vi "P-612 Stage Engine.vi"(0 "Unique Notifier Name":string, 11 "COM Port":string[](array[string])) -> ()   [LabVIEW 2016]
uses:
  Stages Controls/Stage Status.ctl
  Stages Controls/Stage XY Control.ctl
  Stages Controls/Stage Notifier Element.ctl
  Stages Controls/Stage Actions.ctl
panel:
  in  "XY Control":T1={"Left"=FALSE, "Right"=FALSE, "Up"=FALSE, "Down"=FALSE, "Home"=FALSE, "StageStep"=enum."1", "Y"=0.0, "X"=0.0}
  in  "ReInitialize":bool
  in  "Error":bool
  out "Status":T2
  in  "QUIT":bool
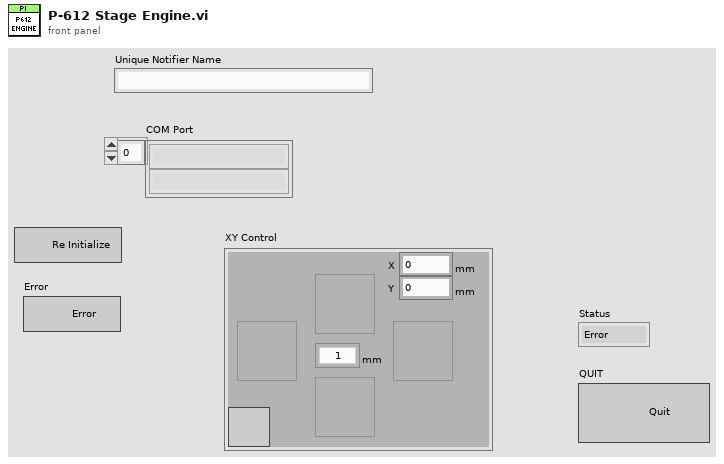
[diagram p1: front panel]
types:
  T1 = typedef "Stage XY Control.ctl" = cluster{"Left":bool, "Right":bool, "Up":bool, "Down":bool, "Home":bool, "StageStep":enum16{"0.01", "0.02", "0.05", "0.1", "0.5", "1", "2", "5", "10", "20", "50", "100", "500", "1000", "2000", "5000"}, "Y":dbl, "X":dbl}
  T2 = typedef "Stage Status.ctl" = enum16{"Error", "Abort", "Busy", "On Target"}
  T3 = typedef "Stage Actions.ctl" = enum16{"Get Position", "MVR", "MOVE", "HALT", "ONTARGET", "ERROR", "REFERENCE", "INIT", "VELOCITY", "STATUS", "EXIT", "HOME", "ZEROPOS", "NANOPOS", "ANALOG", "QUIT"}
  T4 = typedef "Stage Notifier Element.ctl" = cluster{"Action":T3, "Axis":bool[], "Setpoint":dbl[], "Velocity":dbl, "Cmd Recvd?":bool, "Position":dbl[], "Status":T2, "Misc":variant}
  T5 = cluster{"Left":bool, "Right":bool, "Up":bool, "Down":bool, "Home":bool, "StageStep":bool, "Y":bool, "X":bool}
  T6 = enum16{"0.01", "0.02", "0.05", "0.1", "0.5", "1", "2", "5", "10", "20", "50", "100", "500", "1000", "2000", "5000"}
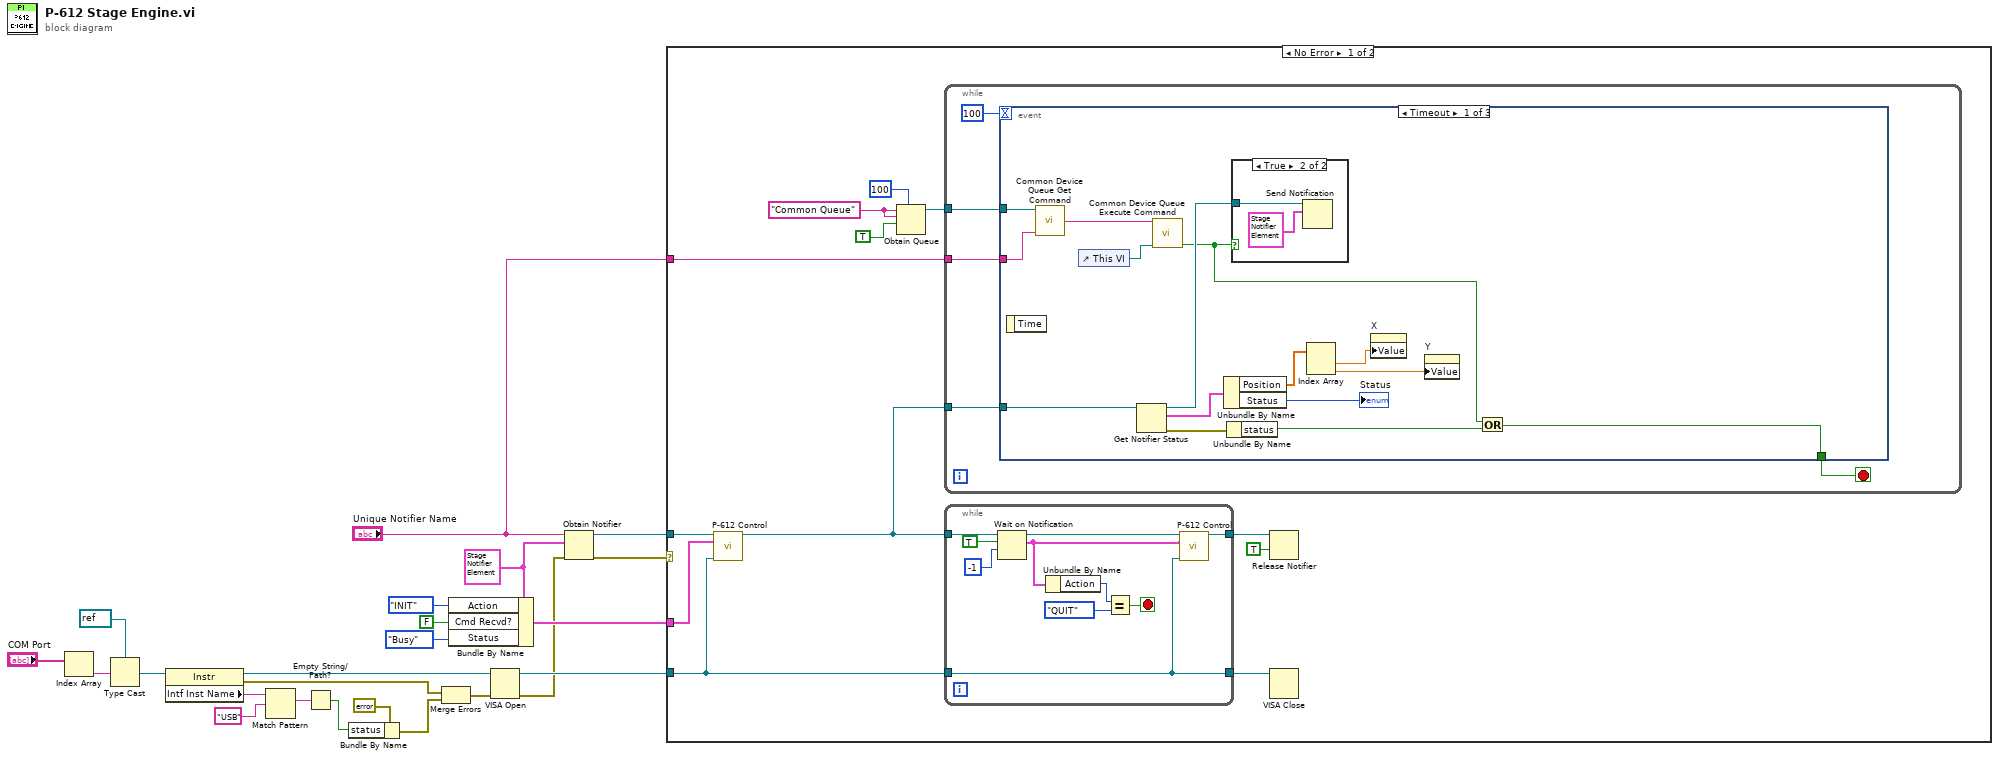
[diagram p0: block diagram]
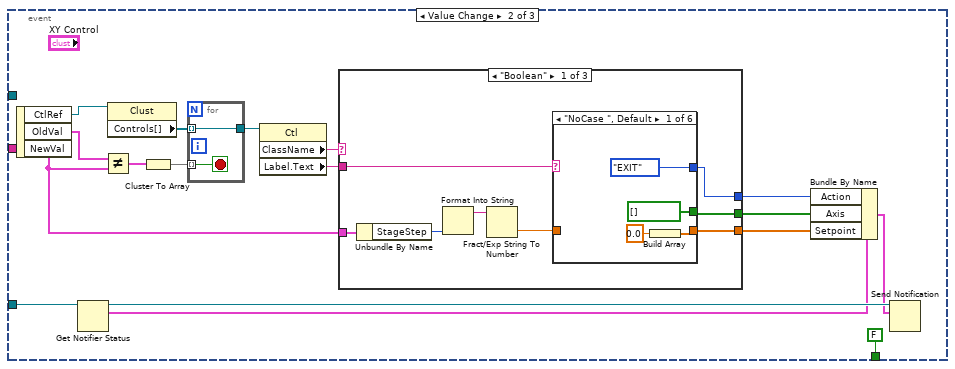
[diagram p3: hidden frame]
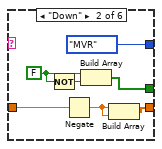
[diagram p4: hidden frame]
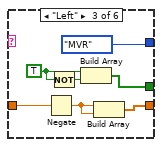
[diagram p5: hidden frame]
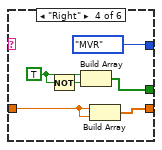
[diagram p6: hidden frame]
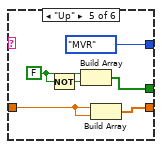
[diagram p7: hidden frame]
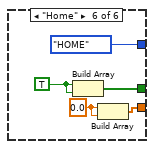
[diagram p8: hidden frame]
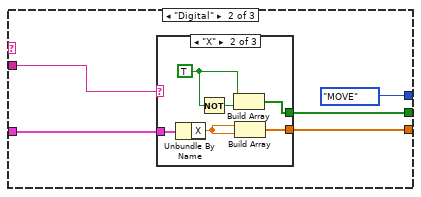
[diagram p9: hidden frame]
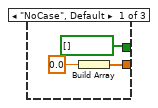
[diagram p10: hidden frame]
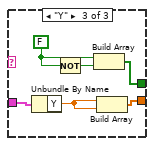
[diagram p11: hidden frame]
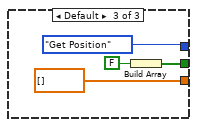
[diagram p12: hidden frame]
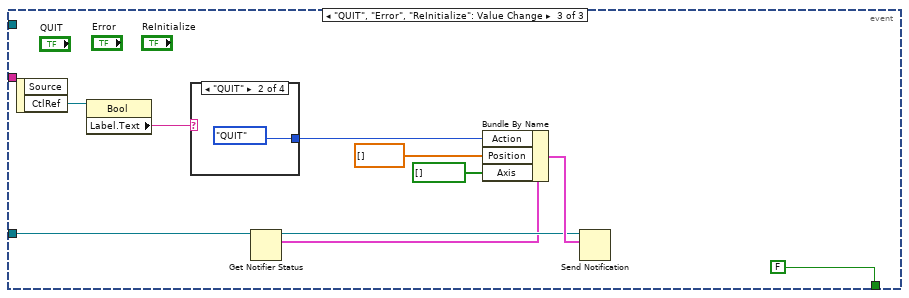
[diagram p13: hidden frame]
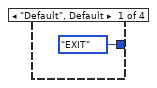
[diagram p14: hidden frame]
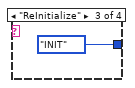
[diagram p15: hidden frame]
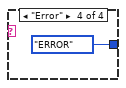
[diagram p16: hidden frame]
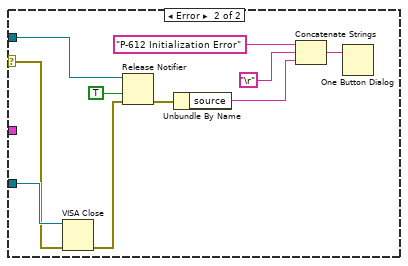
[diagram p17: hidden frame]
diagram:
  w9 = T4 {"Action"=enum."Get Position", "Axis"=[], "Setpoint"=[], "Velocity"=0.5, "Cmd Recvd?"=FALSE, "Position"=[], "Status"=enum."Abort", "Misc"=variant} ("Stage Status")
  n1 = Index Array(array="COM Port") -> (element=w18:string)  [unwired: 1 in]
  n2 = Type Cast(type=refnum<visa-resource-name> refnum ("reference out"), x=w18) -> (*(type *) &x=w16:refnum<visa-resource-name>)
  n3 = property class="Instr"(reference=w16) -> (reference out=w5:refnum<visa-resource-name>, error out=w13:errorcluster, "Intf Inst Name"=w21:string)  [unwired: 1 in]
  n4 = Match Pattern(string=w21, regular expression="USB") -> (match substring=w23:string)  [unwired: 1 in, 3 out]
  n5 = Empty String/Path?(string/path=w23) -> (empty?=w20:bool)
  n6 = Bundle By Name(cluster=errorcluster {"status"=FALSE, "code"=0, "source"=""} ("Error"), "status"=w20) -> (w14:errorcluster)
  n7 = Merge Errors(w13, w14) -> (w4:errorcluster)
  n8 = Bundle By Name(cluster=w9, "Action"=Stage_Actions."INIT", "Cmd Recvd?"=FALSE, "Status"=Stage_Status."Busy") -> (w6:T4)
  n9 = VISA Open(error in (no error)=w4, VISA resource name=w5) -> (VISA resource name=w3:refnum<visa-resource-name>, error out=w2:errorcluster)  [unwired: 3 in]
  n10 = Obtain Notifier(name (unnamed)="Unique Notifier Name", notification data type=w9, error in (no error)=w2) -> (notifier out=w7:refnum<notifier>, error out=w8:errorcluster)  [unwired: 1 in, 1 out]
  n11 = case shown="No Error" w8 {
    selector: w8 -> [_ w168]
    tunnel: w7 -> [w33 w170]
    tunnel: w6 -> [w32 _]
    tunnel: w3 -> [w31 w169]
    tunnel: "Unique Notifier Name" -> [w24 _]
    frame No Error {
      w27 = "Common Queue" ("Unique Notifier Name")
      n12 = call "P-612 Control.vi"("P-612 Notifier"=w33, "Stage Actions"=w32, "VISA In"=w31) -> ("P-612 Notifier (Dup)"=w26:refnum<notifier>)  [unwired: 12 in]
      n13 = Obtain Queue(max queue size (-1, unlimited)=100, name (unnamed)=w27, element data type=w27, create if not found? (T)=TRUE) -> (queue out=w25:refnum<queue>)  [unwired: 1 in, 2 out]
      n14 = while {
        tunnel: w26 -> [w48]
        tunnel: w25 -> [w47]
        tunnel: w24 -> [w46]
        stop <- w49 stop-if-true
        n15 = event shown="[0] Timeout" {
          selector: _ -> [_ _ _]
          dyn-events: _ -> [_ _ _]
          timeout: 100 -> [_ _ _]
          tunnel: [w52 FALSE ("status") FALSE ("status")] -> w49
          tunnel: w48 -> [w59 w68 w154]
          tunnel: w47 -> [w56 _ _]
          tunnel: w46 -> [w55 _ _]
          event Timeout {
            n16 = event-data() -> ()  [unwired: 1 in, 1 out]
            n17 = call "Common Device Queue Get Command.vi"("Common Queue"=w56, "Notifier Name"=w55) -> ("Command"=w57:string)  [unwired: 12 in, 1 out]
            n18 = control-ref of="This VI"() -> (w58:refnum<vi>)
            n19 = Get Notifier Status(notifier=w59) -> (notifier out=w54:refnum<notifier>, current notification=w65:T4, error out=w63:errorcluster)  [unwired: 1 in, 2 out]
            n20 = call "Common Device Queue Execute Command.vi"("Common Command"=w57, "VI Refnum"=w58) -> ("Quit?"=w51:bool)  [unwired: 12 in, 1 out]
            n21 = Unbundle By Name(w65) -> ("Position"=w64:dbl[], "Status"=→"Status":T2)
            n22 = Unbundle By Name(w63) -> ("status"=w53:bool)
            n23 = case shown="True" w51 {
              tunnel: w54 -> [_ w67]
              frame False {
              }
              frame True {
                n24 = Send Notification(notification=T4 {"Action"=enum."QUIT", "Axis"=[], "Setpoint"=[], "Velocity"=0.5, "Cmd Recvd?"=FALSE, "Position"=[], "Status"=enum."Error", "Misc"=variant} ("Stage Status"), notifier=w67) -> ()  [unwired: 1 in, 2 out]
              }
            }
            n25 = Index Array(array=w64) -> (element #1=w61:dbl, element #2=w60:dbl)  [unwired: 2 in]
            n26 = property on="X" class="DigNum (strict)"("Value"=w61) -> ()  [unwired: 2 in, 2 out]
            n27 = property on="Y" class="DigNum (strict)"("Value"=w60) -> ()  [unwired: 2 in, 2 out]
            n28 = Or(x=w51, y=w53) -> (x .or. y?=w52:bool)
          }
          event Value Change {
            n29 = event-data() -> ("CtlRef"=w74:refnum<vi>, "OldVal"=w73:T1, "NewVal"=w72:T1)  [unwired: 1 in]
            n30 = Get Notifier Status(notifier=w68) -> (notifier out=w83:refnum<notifier>, current notification=w82:T4)  [unwired: 1 in, 3 out]
            n31 = Not Equal?(x=w73, y=w72) -> (x != y?=w80:T5)
            n32 = property class="Clust"(reference=w74) -> ("Controls[]"=w78:refnum<vi>[])  [unwired: 1 in, 2 out]
            n33 = Cluster To Array(cluster=w80) -> (array=w79:bool[])
            n34 = for {
              tunnel: w79 -> [w153] mode=indexing
              tunnel: [w152] -> w77
              tunnel: w78 -> [w152] mode=indexing
              stop <- w153 stop-if-true
            }
            n35 = property class="Ctl"(reference=w77) -> ("ClassName"=w76:string, "Label.Text"=w75:string)  [unwired: 1 in, 2 out]
            n36 = case shown="\"Boolean\"" w76 {
              tunnel: w72 -> [w92 w131 _]
              tunnel: w75 -> [w86 w132 _]
              tunnel: [w88 w130 dbl[] []] -> w71
              tunnel: [w89 w129 w150] -> w70
              tunnel: [w87 Stage_Actions."MOVE" ("Action") Stage_Actions."Get Position" ("Action")] -> w69
              frame "Boolean" {
                n37 = Unbundle By Name(w92) -> ("StageStep"=w90:T6)
                n38 = Format Into String(w90) -> (resulting string=w91:string)  [unwired: 3 in, 1 out]
                n39 = Fract/Exp String To Number(string=w91) -> (number=w85:dbl)  [unwired: 3 in, 1 out]
                n40 = case shown="\"NoCase \", Default" w86 {
                  tunnel: [w94 w99 w106 w113 w119 w125] -> w88
                  tunnel: [bool[] [] w100 w107 w114 w120 w127] -> w89
                  tunnel: w85 -> [_ w103 w110 w112 w118 _]
                  tunnel: [Stage_Actions."EXIT" ("Action") Stage_Actions."MVR" ("Action") Stage_Actions."MVR" ("Action") Stage_Actions."MVR" ("Action") Stage_Actions."MVR" ("Action") Stage_Actions."HOME" ("Action")] -> w87
                  frame "NoCase ", Default {
                    n41 = Build Array(0.0) -> (w94:dbl[])
                  }
                  frame "Down" {
                    w101 = FALSE
                    n42 = Not(x=w101) -> (.not. x?=w102:bool)
                    n43 = Negate(x=w103) -> (-x=w98:dbl)
                    n44 = Build Array(w101, w102) -> (w100:bool[])
                    n45 = Build Array(w98, w98) -> (w99:dbl[])
                  }
                  frame "Left" {
                    w108 = TRUE
                    n46 = Negate(x=w110) -> (-x=w105:dbl)
                    n47 = Not(x=w108) -> (.not. x?=w109:bool)
                    n48 = Build Array(w108, w109) -> (w107:bool[])
                    n49 = Build Array(w105, w105) -> (w106:dbl[])
                  }
                  frame "Right" {
                    w115 = TRUE
                    n50 = Not(x=w115) -> (.not. x?=w116:bool)
                    n51 = Build Array(w115, w116) -> (w114:bool[])
                    n52 = Build Array(w112, w112) -> (w113:dbl[])
                  }
                  frame "Up" {
                    w121 = FALSE
                    n53 = Not(x=w121) -> (.not. x?=w122:bool)
                    n54 = Build Array(w121, w122) -> (w120:bool[])
                    n55 = Build Array(w118, w118) -> (w119:dbl[])
                  }
                  frame "Home" {
                    w124 = 0.0
                    w126 = TRUE
                    n56 = Build Array(w126, w126) -> (w127:bool[])
                    n57 = Build Array(w124, w124) -> (w125:dbl[])
                  }
                }
              }
              frame "Digital" {
                n58 = case shown="\"X\"" w132 {
                  tunnel: [bool[] [] w140 w145] -> w129
                  tunnel: w131 -> [_ w139 w144]
                  tunnel: [w133 w138 w143] -> w130
                  frame "NoCase", Default {
                    n59 = Build Array(0.0 ("Y axis (mm)")) -> (w133:dbl[])
                  }
                  frame "X" {
                    w141 = TRUE
                    n60 = Unbundle By Name(w139) -> ("X"=w137:dbl)
                    n61 = Not(x=w141) -> (.not. x?=w136:bool)
                    n62 = Build Array(w141, w136) -> (w140:bool[])
                    n63 = Build Array(w137, w137) -> (w138:dbl[])
                  }
                  frame "Y" {
                    w147 = FALSE
                    n64 = Unbundle By Name(w144) -> ("Y"=w142:dbl)
                    n65 = Not(x=w147) -> (.not. x?=w146:bool)
                    n66 = Build Array(w147, w146) -> (w145:bool[])
                    n67 = Build Array(w142, w142) -> (w143:dbl[])
                  }
                }
              }
              frame Default {
                n68 = Build Array(FALSE) -> (w150:bool[])
              }
            }
            n69 = Bundle By Name(cluster=w82, "Action"=w69, "Axis"=w70, "Setpoint"=w71) -> (w81:T4)
            n70 = Send Notification(notification=w81, notifier=w83) -> ()  [unwired: 1 in, 2 out]
          }
          event "QUIT", "Error", "ReInitialize": Value Change {
            n71 = event-data() -> ("CtlRef"=w157:refnum<vi>)  [unwired: 1 in, 1 out]
            n72 = property class="Bool"(reference=w157) -> ("Label.Text"=w156:string)  [unwired: 1 in, 2 out]
            n73 = case shown="\"QUIT\"" w156 {
              tunnel: [Stage_Actions."EXIT" ("Action") Stage_Actions."QUIT" ("Action") Stage_Actions."INIT" ("Action") Stage_Actions."ERROR" ("Action")] -> w155
              frame "Default", Default {
              }
              frame "QUIT" {
              }
              frame "ReInitialize" {
              }
              frame "Error" {
              }
            }
            n74 = Get Notifier Status(notifier=w154) -> (notifier out=w159:refnum<notifier>, current notification=w158:T4)  [unwired: 1 in, 3 out]
            n75 = Bundle By Name(cluster=w158, "Action"=w155, "Position"=dbl[] [], "Axis"=bool[] []) -> (w160:T4)
            n76 = Send Notification(notification=w160, notifier=w159) -> ()  [unwired: 1 in, 2 out]
          }
        }
      }
      n77 = while {
        tunnel: [w38] -> w34
        tunnel: w26 -> [w40]
        tunnel: w31 -> [w37]
        tunnel: [w37] -> w30
        stop <- w45 stop-if-true
        n78 = Wait on Notification(notifier=w40, ignore previous (F)=TRUE, timeout in ms (-1)=-1) -> (notifier out=w39:refnum<notifier>, notification=w36:T4)  [unwired: 1 in, 2 out]
        n79 = Unbundle By Name(w36) -> ("Action"=w42:T3)
        n80 = Equal?(x=w42, y=Stage_Actions."QUIT") -> (x = y?=w45:bool)
        n81 = call "P-612 Control.vi"("P-612 Notifier"=w39, "Stage Actions"=w36, "VISA In"=w37) -> ("P-612 Notifier (Dup)"=w38:refnum<notifier>)  [unwired: 12 in]
      }
      n82 = Release Notifier(notifier=w34, force destroy? (F)=TRUE) -> ()  [unwired: 1 in, 3 out]
      n83 = VISA Close(VISA resource name=w30) -> ()  [unwired: 1 in, 1 out]
    }
    frame Error {
      n84 = VISA Close(VISA resource name=w169, error in (no error)=w168) -> (error out=w171:errorcluster)
      n85 = Release Notifier(notifier=w170, force destroy? (F)=TRUE, error in (no error)=w171) -> (error out=w176:errorcluster)  [unwired: 2 out]
      n86 = Unbundle By Name(w176) -> ("source"=w173:string)
      n87 = Concatenate Strings("P-612 Initialization Error", "\r", w173) -> (w172:string)
      n88 = One Button Dialog(message=w172) -> ()  [unwired: 1 in, 1 out]
    }
  }
